vi "Size.vi"(8 "error in (no error)":errorcluster, 11 "Double Array in":refnum<class "Double Array.lvclass">) -> (0 "error out":errorcluster, 2 "Size":i32, 3 "Double Array out":refnum<class "Double Array.lvclass">)   [LabVIEW 2020, in "Data.lvlib" / "Double Array.lvclass"]
doc: "Return the size of the generic data element."
uses:
  Double Array.lvclass
  Double Array.lvclass/Double Array.ctl
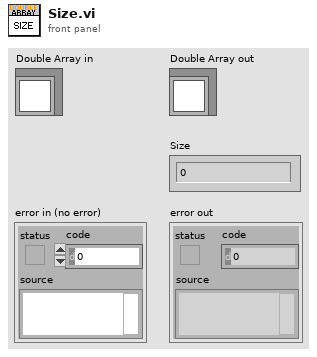
[diagram p1: front panel]
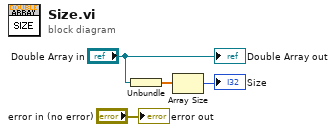
[diagram p0: block diagram]
diagram:
  n1 = Unbundle("Double Array in") -> (w2:dbl[])
  n2 = Array Size(array=w2) -> (size(s)=→"Size":i32)
  "error out" <- "error in (no error)"
  "Double Array out" <- "Double Array in"
